vi "CAN Jaguar Sync Update.vi"(8 "error in (no error)":errorcluster, 10 "bit mask (FF)":u8[](array[numeric])=[255] format="%.0x") -> (0 "error out":errorcluster)   [LabVIEW 2009, in "CAN.lvlib"]
doc: "Sends sync command to the CAN network.\n\nUse bit mask to determine groups to synchronize. By default synchronizes all 8 groups (bitmask 0xFF)"
uses:
  CAN.lvlib
  SubVIs/CAN System Message IDs.ctl
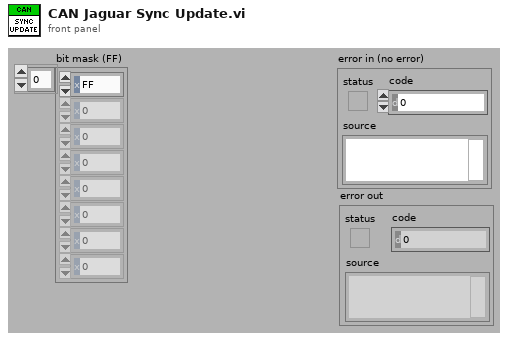
[diagram p1: front panel]
types:
  T1 = typedef "CAN.lvlib/CAN System Message IDs.ctl" = u32
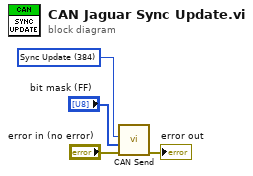
[diagram p0: block diagram]
diagram:
  w2 = T1 384 items=["Device Assignment"=128, "Device Query"=2147483840, "Sync Update"=384, "Firmware Update"=448, "Firmware Version"=2147484160, "Enumerate"=576, "Heartbeat"=320] ("CAN System Message IDs")
  n1 = call "CAN Send.vi"("error in (no error)"="error in (no error)", "data"="bit mask (FF)", "messageID"=w2) -> ("error out"=→"error out":errorcluster)  [unwired: 8 in]
